vi "Value adder.vi"(2 "Array":i16[](array[numeric]), 3 "Enum":enum16{"FWD", "CL", "CT", "Ar", "O2", "Timer"}(ring), 4 "value":i32, 5 "Max Limit":i16) -> (0 "output array":i16[](array[numeric]), 1 "Limited value":i16)   [LabVIEW 2023]
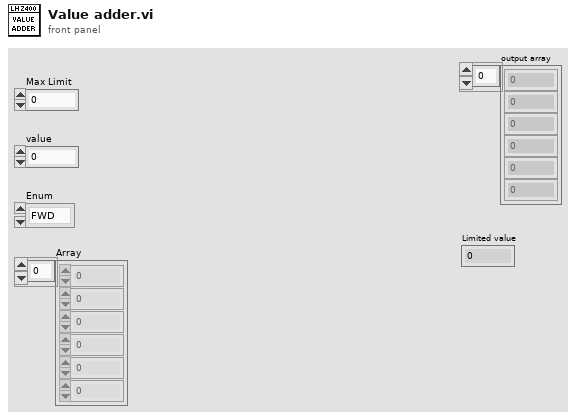
[diagram p1: front panel]
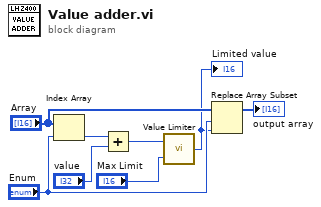
[diagram p0: block diagram]
diagram:
  n1 = Index Array(array="Array", index="Enum") -> (element=w2:i16)
  n2 = Add(x=w2, y="value") -> (x+y=w4:i32)
  n3 = call "Value Limiter.vi"("Max Limit"="Max Limit", "Value"=w4) -> ("Limited value"=w6:i16)
  "Limited value" <- w6
  n4 = Replace Array Subset(array="Array", new element=w6, index="Enum") -> (→"output array":i16[])
